vi "Main.vi"() -> ()   [LabVIEW 2015]
doc: "The myRIO Project template acquires acceleration data from the onboard accelerometer and displays the changes of acceleration values in a waveform chart."
uses:
  <vilib>/myRIO/Common/Instrument Driver Framework/Utilities/typedefs/Generic FPGA Reference.ctl
  <vilib>/myRIO/Common/Instrument Driver Framework/Utilities/typedefs/myRIO v1.0 Reference.ctl
  <vilib>/myRIO/Common/Instrument Driver Framework/Utilities/typedefs/Hardware Version Enum.ctl
  <vilib>/myRIO/Common/Instrument Driver Framework/Utilities/typedefs/myRIO Generic Hardware Reference.ctl
  <vilib>/myRIO/Common/Instrument Driver Framework/Utilities/vis/Is FPGA Ref Available.vi
  <vilib>/userdefined/High Color/nirio_resource_hc.ctl
  <vilib>/myRIO/Instrument Drivers/Onboard IO/PWM/typedefs/PWM Configuration.ctl
  <vilib>/myRIO/Instrument Drivers/Onboard IO/PWM/PWM.lvlib
  <vilib>/myRIO/Common/Instrument Driver Framework/myRIO v1.0/PWM/typedefs/PWM Channels Enum.ctl
  <vilib>/myRIO/Instrument Drivers/Onboard IO/PWM/typedefs/PWM Reference.ctl
  <vilib>/myRIO/Instrument Drivers/Onboard IO/PWM/vis/Set Duty Cycle and Frequency.vi
  <vilib>/myRIO/Common/Instrument Driver Framework/myRIO v1.0/PWM/vis/myRIO v1.1 Open PWM.vi
  <vilib>/myRIO/Instrument Drivers/Onboard IO/PWM/vis/myRIO PWM Open.xnode
  <vilib>/myRIO/Express VI/Onboard IO/PWM/PWM Express VI.xnode
  <vilib>/Instr/_visa.llb/VISA Configure Serial Port (Instr).vi
panel:
  in  "Stop (F)":bool
  out "Image Out":T1(plugin-control)
  out "Latitude [deg]":string
  out "Longitude":string
  out "Number of satellites in use":dbl
  out "NMEA Sentances":string
  out "Command Number":i32
  out "Y Value":i32
  out "X Value":i32
  in  "ON duty cycle":dbl
  in  "OFF duty cycle":dbl
  in  "Duty Cycle 3":dbl=0.5
  in  "Duty Cycle 2":dbl=0.5
  in  "Duty Cycle 1":dbl=0.5
  in  "Frequency [Hz]":dbl=1000.0
  in  "Desired Position":dbl[](array[numeric])
  in  "Blimp Orientation":dbl
  in  "Desired Orientation":dbl
  in  "NAVIGATION STOP":bool
  in  "Blimp Postion":dbl[](array[numeric])
  out "BLIMP POSITION":cluster{"Y":dbl[], "Y":dbl[]}[](graph)
  in  "STOP":bool
  # "ACTUAL STATES OF BLIMP"
  # "DESIRED STATES OF BLIMP"
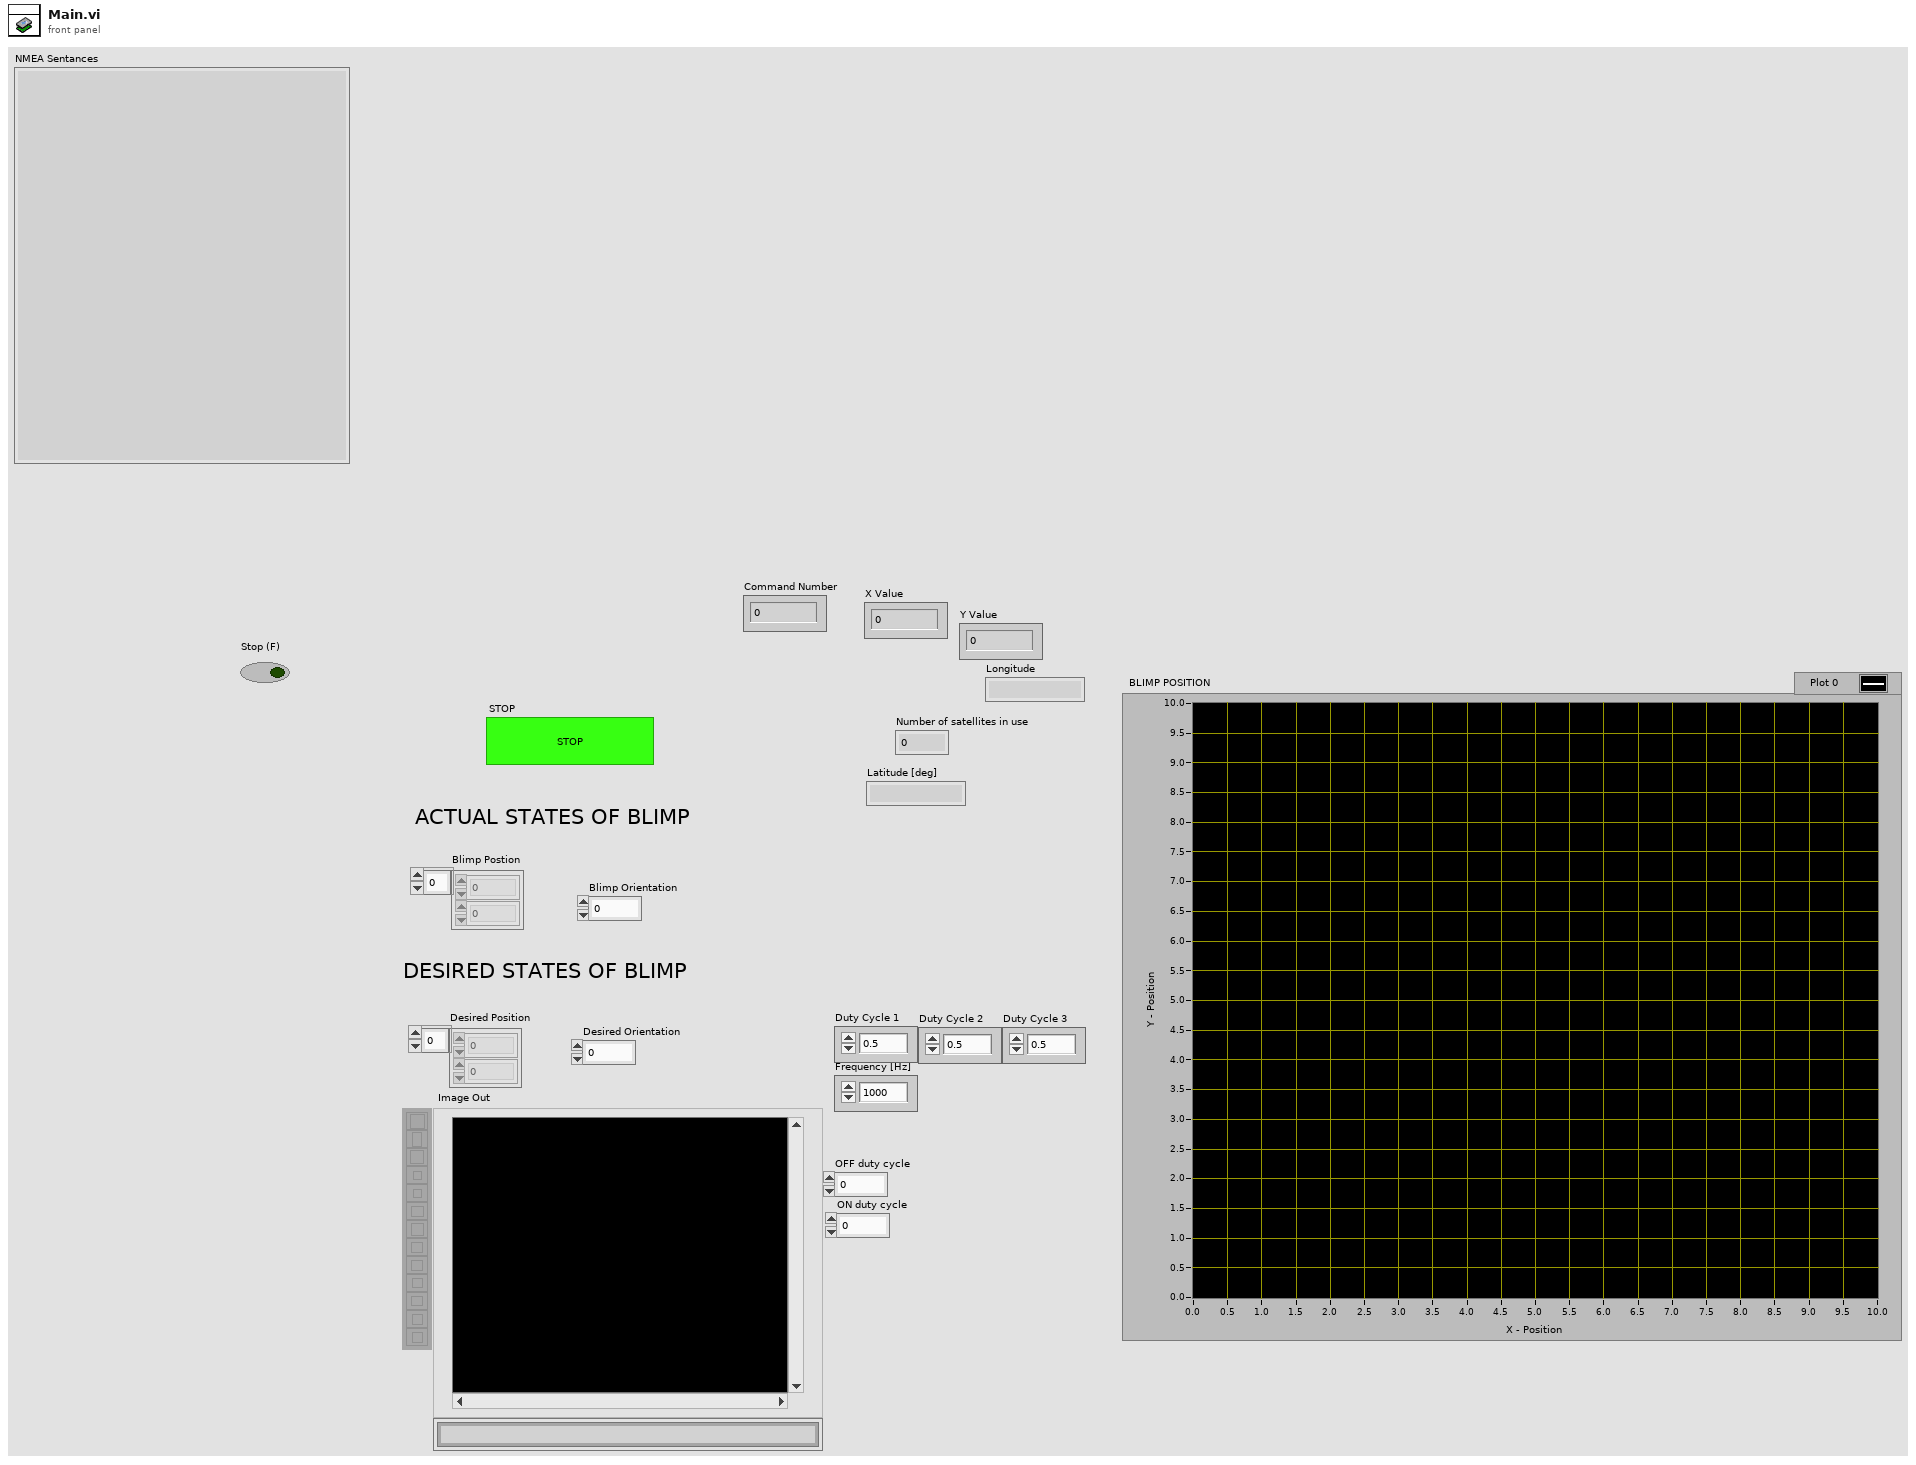
[diagram p1: front panel]
types:
  T1 = typedef "IMAQ Image.ctl" = refnum<image>
  T2 = typedef "PWM.lvlib/PWM Reference.ctl" = cluster{"myRIO Reference":T3, "PWM Channels Enum":T7, "PWM Configuration":T8}
  T3 = typedef "myRIO Generic Hardware Reference.ctl" = cluster{"myRIO Model":T4, "myRIO Hardware Reference":T5}
  T4 = typedef "Hardware Version Enum.ctl" = enum16{"Unknown", "myRIO-1900", "myRIO-1950", "roboRIO"}
  T5 = typedef "myRIO v1.0 Reference.ctl" = cluster{"Generic FPGA Reference":T6, "Allow multiple opens":bool}
  T6 = typedef "Generic FPGA Reference.ctl" = refnum<k20>
  T7 = typedef "PWM Channels Enum.ctl" = enum16{"Not Connected", "C/PWM0", "C/PWM1", "A/PWM0", "A/PWM1", "A/PWM2", "B/PWM0", "B/PWM1", "B/PWM2", "PWM/PWM0", "PWM/PWM1", "PWM/PWM2", "PWM/PWM3", "PWM/PWM4", "PWM/PWM5", "PWM/PWM6", "PWM/PWM7", "PWM/PWM8", "PWM/PWM9"}
  T8 = typedef "PWM.lvlib/PWM Configuration.ctl" = cluster{"Frequency":dbl, "Duty Cycle":dbl}
  T9 = typedef "nirio_resource_hc.ctl" = tag
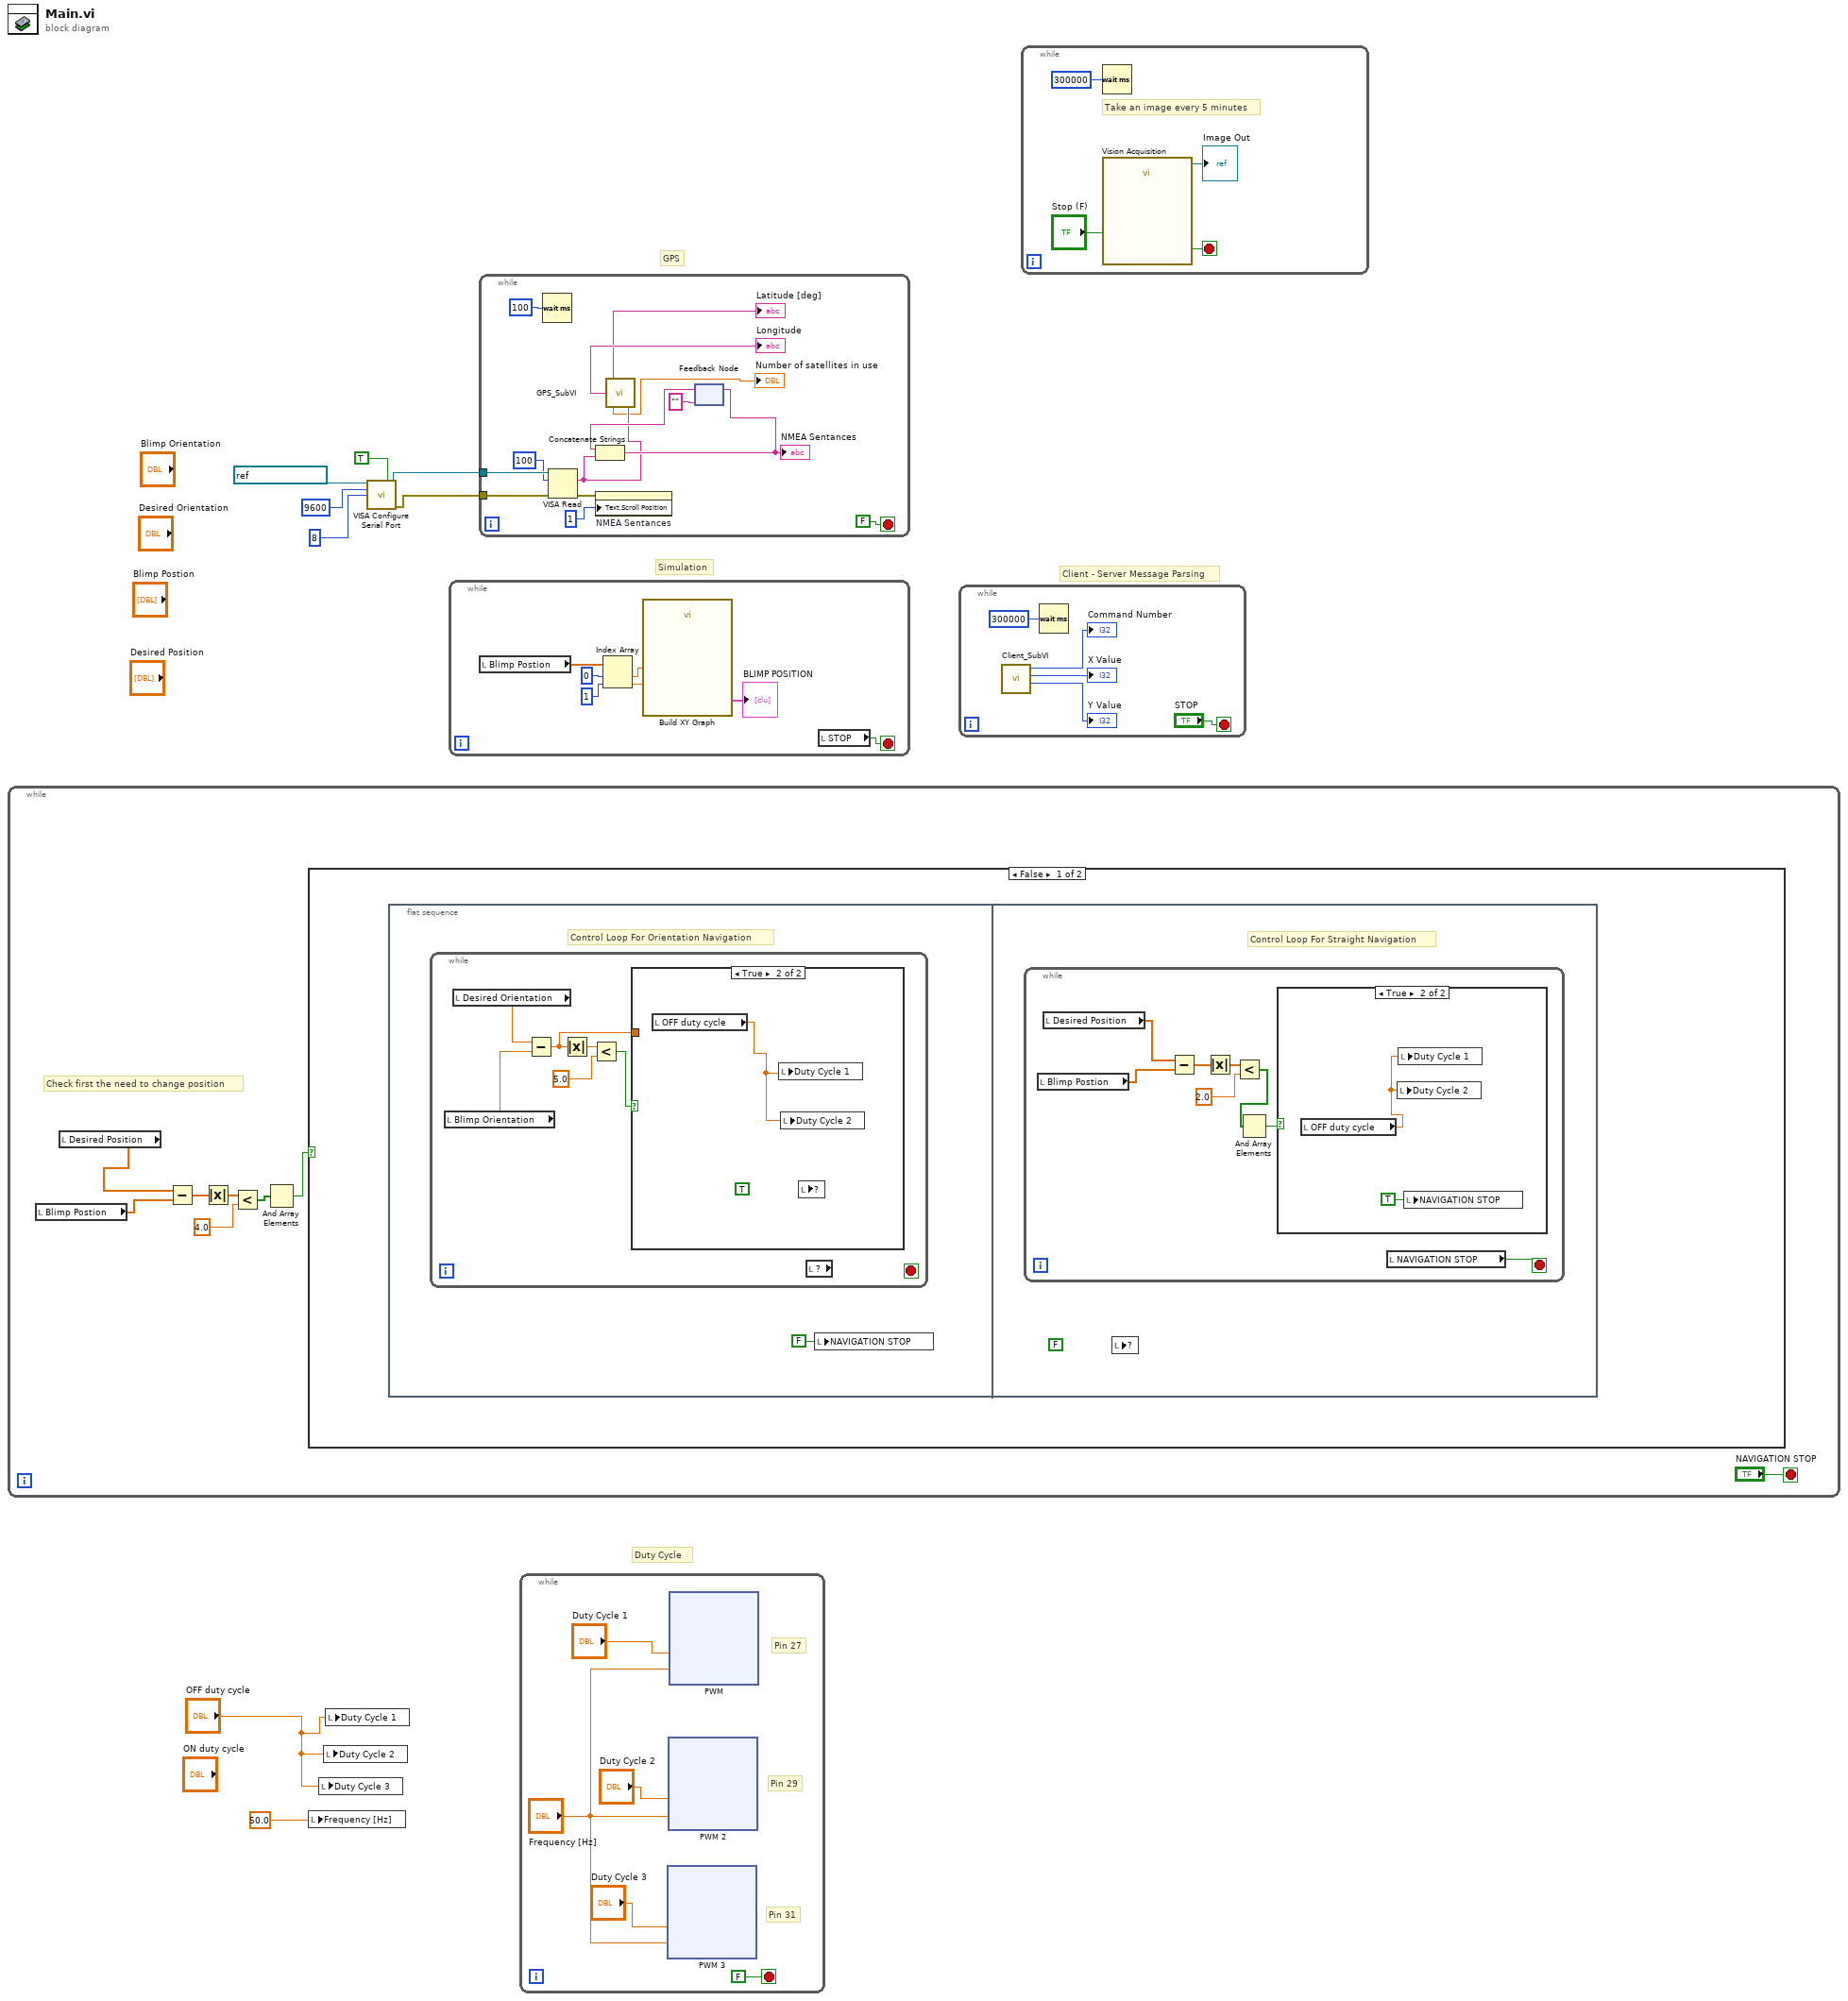
[diagram p0: block diagram]
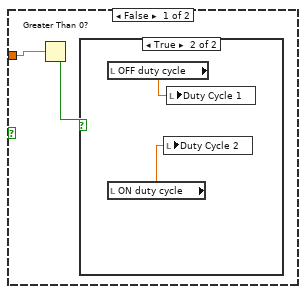
[diagram p2: hidden frame]
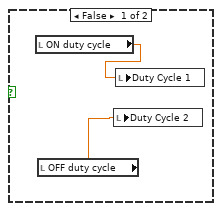
[diagram p3: hidden frame]
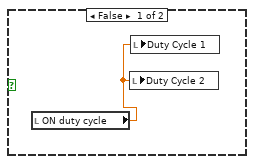
[diagram p4: hidden frame]
diagram:
  # "GPS"
  # "Duty Cycle"
  # "Simulation"
  # "Client - Server Message Parsing"
  n1 = while {
    stop <- "NAVIGATION STOP" stop-if-true
    # "Check first the need to change position"
    n2 = local read "Blimp Postion"() -> (w12:dbl[])
    n3 = local read "Desired Position"() -> (w11:dbl[])
    n4 = Subtract(x=w11, y=w12) -> (x-y=w13:dbl[])
    n5 = Absolute Value(x=w13) -> (abs(x)=w14:dbl[])
    n6 = Less?(x=w14, y=4.0) -> (x < y?=w16:bool[])
    n7 = And Array Elements(Boolean array=w16) -> (logical AND=w10:bool)
    n8 = case shown="False" w10 {
      frame False {
        n9 = flat-sequence {
          frame #0 {
            # "Control Loop For Orientation Navigation"
            n10 = while {
              stop <- _ stop-if-true
              n11 = local read "Blimp Orientation"() -> (w20:dbl)
              n12 = local read "Desired Orientation"() -> (w21:dbl)
              n13 = Subtract(x=w21, y=w20) -> (x-y=w19:dbl)
              n14 = Absolute Value(x=w19) -> (abs(x)=w22:dbl)
              n15 = Less?(x=w22, y=5.0) -> (x < y?=w18:bool)
              n16 = case shown="True" w18 {
                tunnel: w19 -> [w25 _]
                frame False {
                  n17 = Greater Than 0?(x=w25) -> (x > 0?=w24:bool)
                  n18 = case shown="True" w24 {
                    frame False {
                      n19 = local read "ON duty cycle"() -> (w27:dbl)
                      n20 = local read "OFF duty cycle"() -> (w26:dbl)
                      n21 = local write "Duty Cycle 2"(w26) -> ()
                      n22 = local write "Duty Cycle 1"(w27) -> ()
                    }
                    frame True {
                      n23 = local read "OFF duty cycle"() -> (w29:dbl)
                      n24 = local read "ON duty cycle"() -> (w28:dbl)
                      n25 = local write "Duty Cycle 2"(w28) -> ()
                      n26 = local write "Duty Cycle 1"(w29) -> ()
                    }
                  }
                }
                frame True {
                  (unwired) TRUE ("ROTATION STOP")
                  n27 = local read "OFF duty cycle"() -> (w30:dbl)
                  n28 = local write "Duty Cycle 1"(w30) -> ()
                  n29 = local write "Duty Cycle 2"(w30) -> ()
                  n30 = local read item#-1() -> ()  [unwired: 1 in]
                }
              }
              n31 = local read item#-1() -> ()  [unwired: 1 out]
            }
            n32 = local write "NAVIGATION STOP"(FALSE ("NAVIGATION STOP")) -> ()
          }
          frame #1 {
            (unwired) FALSE ("ROTATION STOP")
            # "Control Loop For Straight Navigation"
            n33 = while {
              stop <- w31 stop-if-true
              n34 = local read "Blimp Postion"() -> (w38:dbl[])
              n35 = local read "Desired Position"() -> (w32:dbl[])
              n36 = Subtract(x=w32, y=w38) -> (x-y=w37:dbl[])
              n37 = Absolute Value(x=w37) -> (abs(x)=w36:dbl[])
              n38 = Less?(x=w36, y=2.0) -> (x < y?=w33:bool[])
              n39 = And Array Elements(Boolean array=w33) -> (logical AND=w34:bool)
              n40 = case shown="True" w34 {
                frame False {
                  n41 = local read "ON duty cycle"() -> (w39:dbl)
                  n42 = local write "Duty Cycle 2"(w39) -> ()
                  n43 = local write "Duty Cycle 1"(w39) -> ()
                }
                frame True {
                  n44 = local read "OFF duty cycle"() -> (w41:dbl)
                  n45 = local write "Duty Cycle 2"(w41) -> ()
                  n46 = local write "Duty Cycle 1"(w41) -> ()
                  n47 = local write "NAVIGATION STOP"(TRUE ("NAVIGATION STOP")) -> ()
                }
              }
              n48 = local read "NAVIGATION STOP"() -> (w31:bool)
            }
            n49 = local read item#-1() -> ()  [unwired: 1 in]
          }
        }
      }
      frame True {
      }
    }
  }
  n50 = local write "Frequency [Hz]"(50.0) -> ()
  n51 = local write "Duty Cycle 3"("OFF duty cycle") -> ()
  n52 = local write "Duty Cycle 2"("OFF duty cycle") -> ()
  n53 = local write "Duty Cycle 1"("OFF duty cycle") -> ()
  n54 = call-poly "VISA Configure Serial Port"("VISA resource name"=refnum<visa-resource-name> "ASRL1::INSTR", "Enable Termination\nChar (T)"=TRUE ("Enable Termination\nChar (T)"), "baud rate (9600)"=u32 9600, "data bits (8)"=u16 8) -> ("VISA resource name out"=w4:refnum<visa-resource-name>, "error out"=w3:errorcluster)  [unwired: 10 in]
  n55 = while {
    stop <- w48 stop-if-true
    n56 = local read "Blimp Postion"() -> (w46:dbl[])
    n57 = Index Array(array=w46, index #1=0 ("index"), index #2=1 ("index")) -> (element #1=w43:dbl, element #2=w42:dbl)
    n58 = call "Build XY Graph"("Y Input"=w42, "X Input"=w43) -> ("XY Graph"=→"BLIMP POSITION":cluster{"Y":dbl[], "Y":dbl[]}[])  [unwired: 3 in, 6 out]
    n59 = local read "STOP"() -> (w48:bool)
  }
  n60 = while {
    tunnel: w4 -> [w62]
    tunnel: w3 -> [w61]
    stop <- FALSE stop-if-true
    n61 = Wait (ms)(milliseconds to wait=u32 100) -> ()  [unwired: 1 out]
    n62 = VISA Read(VISA resource name=w62, byte count=u32 100, error in (no error)=w61) -> (read buffer=w52:string, error out=w56:errorcluster)  [unwired: 2 out]
    n63 = property on="NMEA Sentances" class="Str"(error in=w56, "Text.Scroll Position"=u32 1) -> ()  [unwired: 1 in, 2 out]
    n64 = call "GPS_SubVI.vi"("read buffer"=w52) -> ("Number of satellites in use"=→"Number of satellites in use":dbl, "Longitude"=→"Longitude":string, "Latitude [deg]"=→"Latitude [deg]":string)
    n65 = feedback #1("") -> (w58:string)
    n66 = Concatenate Strings "Concatenate Strings"(w58, w52) -> (w59:string)
    "NMEA Sentances" <- w59
    n67 = feedback-in #1(w59) -> ()
  }
  n68 = while {
    stop <- FALSE stop-if-true
    # "Pin 31"
    # "Pin 29"
    # "Pin 27"
    n69 = xnode "PWM 3"("Duty Cycle"="Duty Cycle 3", "Frequency [Hz]"="Frequency [Hz]") -> ()  [unwired: 1 in, 1 out]
    n70 = xnode "PWM 2"("Duty Cycle"="Duty Cycle 2", "Frequency [Hz]"="Frequency [Hz]") -> ()  [unwired: 1 in, 1 out]
    n71 = xnode "PWM"("Duty Cycle"="Duty Cycle 1", "Frequency [Hz]"="Frequency [Hz]") -> ()  [unwired: 1 in, 1 out]
  }
  n72 = while {
    stop <- "STOP" stop-if-true
    n73 = call "Client_SubVI.vi"() -> ("Numeric"=→"Y Value":i32, "Numeric 2"=→"X Value":i32, "Numeric 3"=→"Command Number":i32)  [unwired: 9 in]
    n74 = Wait (ms)(milliseconds to wait=u32 300000) -> ()  [unwired: 1 out]
  }
  n75 = while {
    stop <- w179 stop-if-true
    # "Take an image every 5 minutes"
    n76 = Wait (ms)(milliseconds to wait=u32 300000) -> ()  [unwired: 1 out]
    n77 = call "Vision Acquisition"("Stop (F)"="Stop (F)") -> ("Image Out"=→"Image Out":T1, "Stopped"=w179:bool)  [unwired: 24 in, 1 out]
  }
